vi "Double Point CW.vi"() -> ()   [LabVIEW 2020]
uses:
  Labview Library/Libraries/Basic Experiment/CW Results.ctl
  Labview Library/Libraries/Basic Experiment/CW Fit Frequency.ctl
  <vilib>/Math Plots/2D Math Plots/2D Error Bar/2D Error Bar XCtrl/2D Error Bar.xctl
  <vilib>/Math Plots/2D Math Plots/2D Error Bar/2D Error Bar Datatype/2D Error Bar Datatype.lvclass
  Labview Library/Libraries/Basic Experiment/CW settings.ctl
  Labview Library/Libraries/Basic Experiment/AutoTrace Setting For Exp.ctl
  Labview Library/Libraries/HW_LMMR_ASG8100/LMMR ASG/ASG Instructions XControl.xctl
  <vilib>/Analysis/baseanly.llb/Mean (DBL).vi
  <vilib>/Math Plots/2D Math Plots/2D Error Bar/2D Error Bar Datatype/Public/Plot Helper (Fixed).vi
  <vilib>/express/express arith-compare/Formula/XNode/ExpressFormulaBlockNode.xnode
  Labview Library/Libraries/Basic Experiment/Basic Experiment.lvlib
  Labview Library/Libraries/HW_LMMR_ASG8100/LMMR ASG/ASG 8100 Module.lvlib
  Labview Library/Libraries/HW_NI_CTR/NI DAQ Counter/NI DAQ Counter.lvlib
  <vilib>/Analysis/NI_AALBase.lvlib
  Labview Library/Libraries/HW_Rigol_DSG/Rigol Signal Generator Module/Rigol Signal Generator Module.lvlib
panel:
  in  "?":enum32{"CW Sequence", "CW Spectrum CY", "Check"}(tab)=enum."CW Spectrum CY"
  in  "CW seq":T3(xcontrol)=[{"Flags"=[TRUE, FALSE, FALSE, FALSE, FALSE, FALSE, FALSE, FALSE, FALSE, FALSE, FALSE, FALSE, FALSE, FALSE], "Comments"="", "Time"=2e-06, "Loop Config"={"Loop Code"=enum."Continued", "Number of Loop"=0, "End of Loop"=nan, "Loop Info"=""}}, {"Flags"=[TRUE, FALSE, TRUE, FALSE, FALSE, FALSE, FALSE, FALSE, FALSE, FALSE, FALSE, FALSE, FALSE, FALSE], "Comments"="", "Time"=5e-08, "Loop Config"={"Loop Code"=enum."Continued", "Number of Loop"=0, "End of Loop"=nan, "Loop Info"=""}}, {"Flags"=[TRUE, TRUE, FALSE, FALSE, FALSE, FALSE, FALSE, FALSE, FALSE, FALSE, FALSE, FALSE, FALSE, FALSE], "Comments"="", "Time"=5e-05, "Loop Config"={"Loop Code"=enum."Continued", "Number of Loop"=0, "End of Loop"=nan, "Loop Info"=""}}, {"Flags"=[TRUE, FALSE, TRUE, FALSE, FALSE, FALSE, FALSE, FALSE, FALSE, FALSE, FALSE, FALSE, FALSE, FALSE], "Comments"="", "Time"=5e-08, "Loop Config"={"Loop Code"=enum."Continued", "Number of Loop"=0, "End of Loop"=nan, "Loop Info"=""}}, {"Flags"=[TRUE, FALSE, FALSE, FALSE, FALSE, FALSE, FALSE, FALSE, TRUE, FALSE, FALSE, FALSE, FALSE, FALSE], "Comments"="", "Time"=2e-06, "Loop Config"={"Loop Code"=enum."Continued", "Number of Loop"=0, "End of Loop"=nan, "Loop Info"=""}}, {"Flags"=[TRUE, FALSE, TRUE, FALSE, FALSE, FALSE, FALSE, FALSE, FALSE, FALSE, FALSE, FALSE, FALSE, FALSE], "Comments"="", "Time"=5e-08, "Loop Config"={"Loop Code"=enum."Continued", "Number of Loop"=0, "End of Loop"=nan, "Loop Info"=""}}, {"Flags"=[TRUE, FALSE, FALSE, FALSE, FALSE, FALSE, FALSE, FALSE, FALSE, FALSE, FALSE, FALSE, FALSE, FALSE], "Comments"="", "Time"=5e-05, "Loop Config"={"Loop Code"=enum."Continued", "Number of Loop"=0, "End of Loop"=nan, "Loop Info"=""}}, {"Flags"=[TRUE, FALSE, TRUE, FALSE, FALSE, FALSE, FALSE, FALSE, FALSE, FALSE, FALSE, FALSE, FALSE, FALSE], "Comments"="", "Time"=5e-08, "Loop Config"={"Loop Code"=enum."Continued", "Number of Loop"=0, "End of Loop"=nan, "Loop Info"=""}}, {"Flags"=[TRUE, FALSE, FALSE, FALSE, FALSE, FALSE, FALSE, FALSE, FALSE, FALSE, FALSE, FALSE, FALSE, FALSE], "Comments"="", "Time"=2e-06, "Loop Config"={"Loop Code"=enum."Continued", "Number of Loop"=0, "End of Loop"=nan, "Loop Info"=""}}]
  out "Signal and Ref 2":cluster{"Numeric":dbl, "Numeric":dbl}(graph)={"Numeric"=11988.666666666666, "Numeric"=11908.666666666666}
  out "Signal and Ref":cluster{"Numeric":dbl, "Numeric":dbl}(graph)={"Numeric"=12031.333333333334, "Numeric"=11977.333333333332}
  in  "Settings":T4={"Num Pts"=10000, "Start freq"=1367.0, "Stop freq"=1373.0, " dBm"=-7.0, "Ratio \nThre(abs)"=0.03, "AutoTrace Before Exp"=FALSE, "RepoSave"=FALSE, "Peak Num \nLimit "=2, "Loop per Update"=1200, "UpdateTime"=25} {"UpdateTime" format="%.0p"; "Loop per Update" format="%#_6p"}
  in  "AutoTrace Settings":T5={"Ratio"=0.5, "Threshold"=7170.999999999999, "Trace Times"=0, "Max Times"=100, "AutoTrace Status"=enum."Normal"}
  out "Total Time (min)":ext=1062.1593 format="%#.5p"
  out "Readout Result":refnum<class "2D Plot Datatype.lvclass">[](xcontrol) caption="2D Error Bar"
  out "CW Result":T6={"Fit Frequency"={"Fre2"={"Amplitude"=nan, "Position"=nan, "Width"=nan}, "Fre1"={"Amplitude"=nan, "Position"=nan, "Width"=nan}, "Fre3"={"Amplitude"=nan, "Position"=nan, "Width"=nan}, "Background"=0.0}, "Pro"=[], "Error Bar"=[0.009618072395389447, 0.010023899080911879, 0.0099506405925294, 0.010065376148420763, 0.010199717043787939, 0.010260847634534493, 0.010058201169096073, 0.010330373101194222, 0.010347960338142663, 0.010432270152347089, 0.010424891842338956, 0.010339921852896642, 0.01058656495840666, 0.010634567325262224], "Raw Data Path"=path "", "Image Path"=path ""}
  out "Pro Array":dbl[](array[numeric])=[-0.0022504507719500744, 0.003304738238140814, -0.01707959605598075, -0.01598738795963195, -0.00726438373136129, -0.005972380429531077, -0.030821164777634635, -0.009807610308887105, -0.011284996490708799, -0.006280515739338632, -0.0033235649624780983, -0.010049154116550496, 0.006197937645131102, 0.007759603066543885]
  in  "error in (no error)":errorcluster={"status"=FALSE, "code"=1073676294, "source"="VISA Read in YP60.lvlib:Wrap VISA Read.vi:5740004->YP60.lvlib:VISA Set Current.vi:2010003->YP60.lvlib:Set Core.vi->YP60.lvlib:Main.vi"}
  out "error out":errorcluster={"status"=TRUE, "code"=-1073807194, "source"="VISA Write in Rigol Signal Generator Module.lvlib:Stop - CORE.vi->Rigol Signal Generator Module.lvlib:Main.vi->Rigol Signal Generator Module.lvlib:Main.vi.ACBRProxyCaller.FA10008D"}
  # "CW Settings"
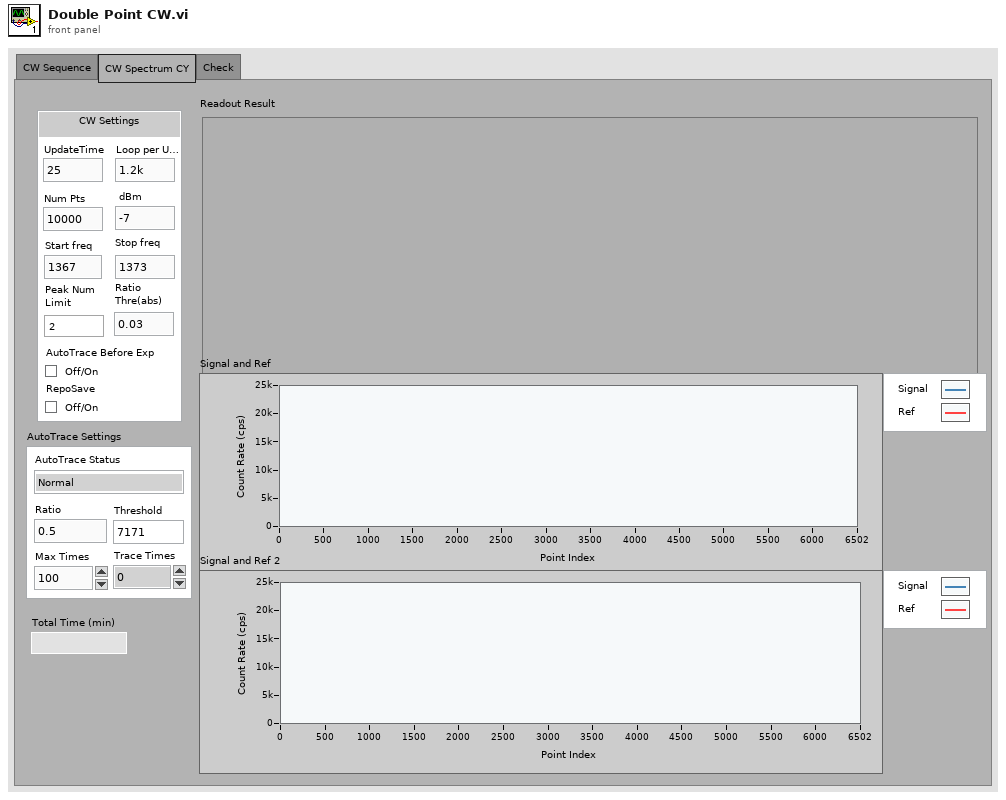
[diagram p1: front panel]
types:
  T1 = typedef "Loop XControl.xctl/Loop Config.ctl" = cluster{"Loop Code":T2, "Number of Loop":i32, "End of Loop":dbl, "Loop Info":string}
  T2 = typedef "Loop XControl.xctl/Loop Code.ctl" = enum16{"Continued", "Loop", "End Loop"}
  T3 = cluster{"Flags":bool[], "Comments":string, "Time":dbl, "Loop Config":T1}[]
  T4 = typedef "Basic Experiment.lvlib/CW settings.ctl" = cluster{"Num Pts":i32, "Start freq":dbl, "Stop freq":dbl, " dBm":dbl, "Ratio \nThre(abs)":dbl, "AutoTrace Before Exp":bool, "RepoSave":bool, "Peak Num \nLimit ":i32, "Loop per Update":u32, "UpdateTime":i32}
  T5 = typedef "Basic Experiment.lvlib/AutoTrace Setting For Exp.ctl" = cluster{"Ratio":dbl, "Threshold":dbl, "Trace Times":i32, "Max Times":i32, "AutoTrace Status":enum16{"Normal", "AutoTrace  Last Loop", "Unintialized"}}
  T6 = typedef "Basic Experiment.lvlib/CW Results.ctl" = cluster{"Fit Frequency":T7, "Pro":dbl[], "Error Bar":dbl[], "Raw Data Path":path, "Image Path":path}
  T7 = typedef "Basic Experiment.lvlib/CW Fit Frequency.ctl" = cluster{"Fre2":cluster{"Amplitude":dbl, "Position":dbl, "Width":dbl}, "Fre1":cluster{"Amplitude":dbl, "Position":dbl, "Width":dbl}, "Fre3":cluster{"Amplitude":dbl, "Position":dbl, "Width":dbl}, "Background":dbl}
  T8 = cluster{"Sweep Amplitude (V)":dbl, "Freq Start (Hz)":dbl, "Freq Stop (Hz)":dbl, "Num of Point":i32}
  T9 = enum16{"Normal", "AutoTrace  Last Loop", "Unintialized"}
  T10 = enum16{"open", "open or create", "create or replace", "create", "open (read-only)"}
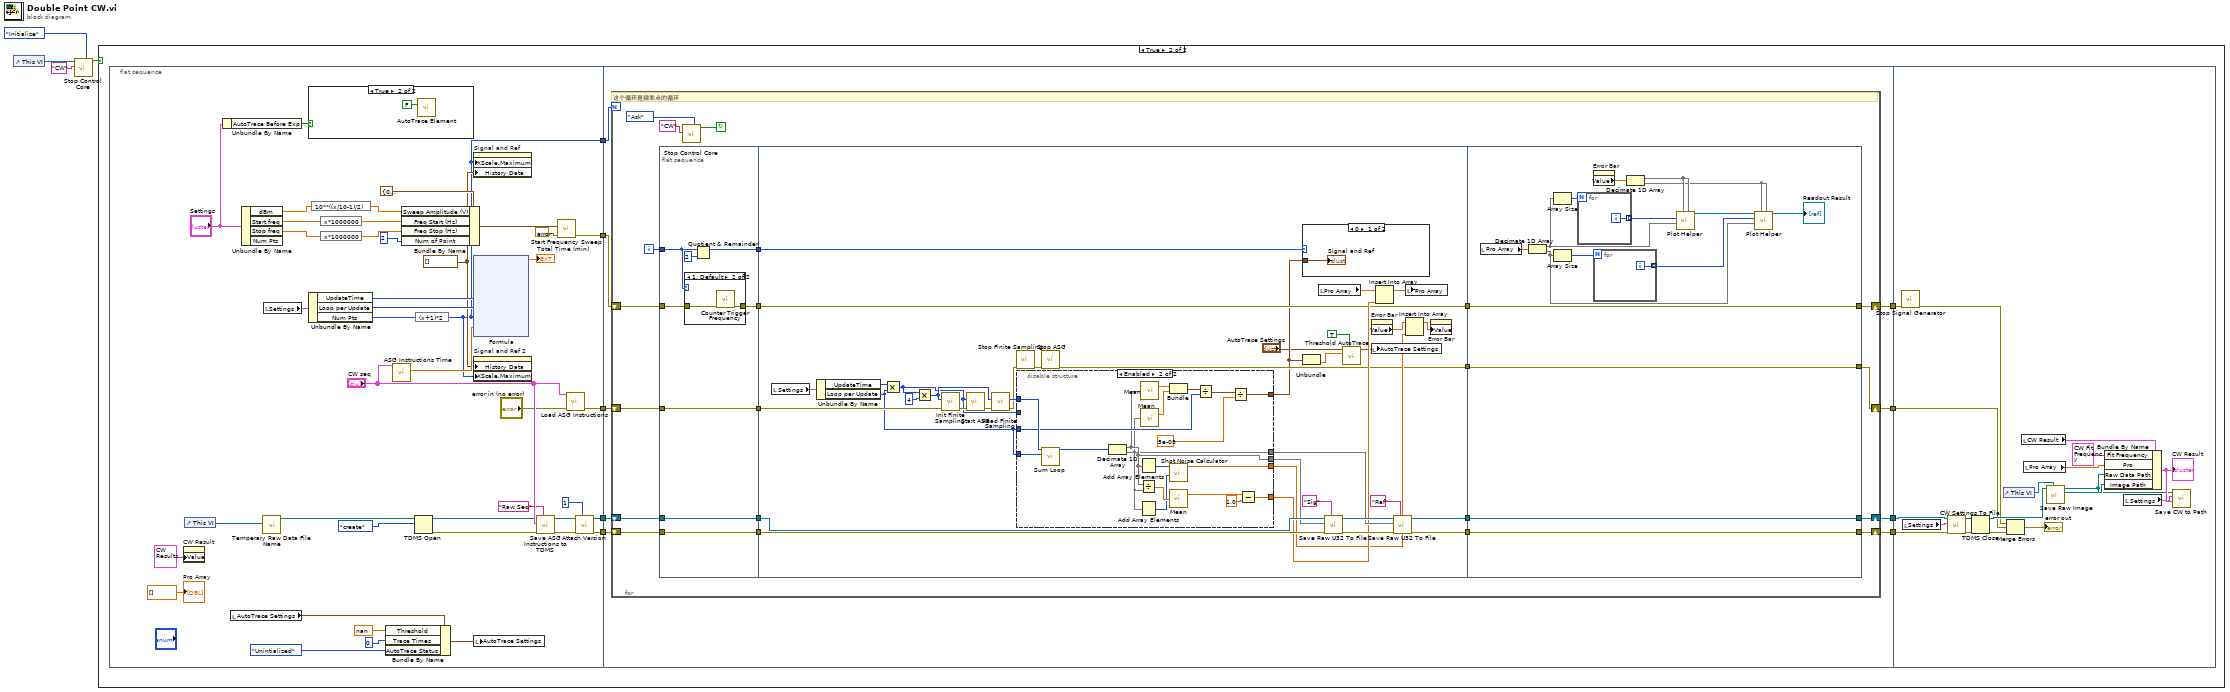
[diagram p0: block diagram]
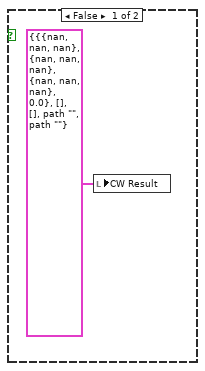
[diagram p2: hidden frame]
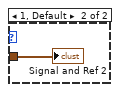
[diagram p5: hidden frame]
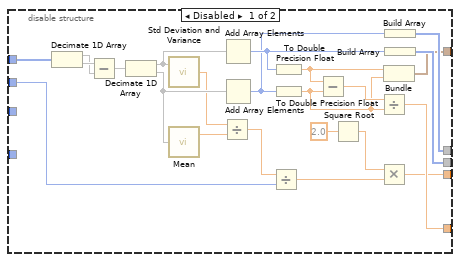
[diagram p6: hidden frame]
diagram:
  n1 = control-ref of="This VI"() -> (w3:refnum<vi>)
  n2 = call "Stop Control Core.vi"("Mode"=enum16{"Ask", "Initialize"}."Initialize", "Program Name"="CW", "VI Ref"=w3) -> ("Continue Sign(Continue:True)"=w1:bool)  [unwired: 8 in]
  n3 = case shown="True" w1 {
    frame False {
      n4 = local write "CW Result"(T6 {"Fit Frequency"={"Fre2"={"Amplitude"=nan, "Position"=nan, "Width"=nan}, "Fre1"={"Amplitude"=nan, "Position"=nan, "Width"=nan}, "Fre3"={"Amplitude"=nan, "Position"=nan, "Width"=nan}, "Background"=0.0}, "Pro"=[], "Error Bar"=[], "Raw Data Path"=path "", "Image Path"=path ""} ("CW Result")) -> ()
    }
    frame True {
      n5 = flat-sequence {
        tunnel: [w35] -> w11
        tunnel: [w39] -> w10
        tunnel: [w38] -> w9
        tunnel: [w37] -> w8
        tunnel: [w16] -> w6
        tunnel: [w80] -> w14
        tunnel: [w79] -> w13
        tunnel: [w78] -> w12
        tunnel: w11 -> [w77]
        tunnel: w10 -> [w76]
        tunnel: w9 -> [w75]
        tunnel: w8 -> [w74]
        tunnel: [w73] -> w7
        tunnel: w6 -> [w72]
        tunnel: w14 -> [w229]
        tunnel: w13 -> [w228]
        tunnel: w12 -> [w216]
        tunnel: w7 -> [w214]
        frame #0 {
          w17 = cluster{"Signal":dbl, "Ref":dbl}[] [] ("History Data")
          n6 = property on="CW Result" class="Clust (strict)"("Value"=T6 {"Fit Frequency"={"Fre2"={"Amplitude"=nan, "Position"=nan, "Width"=nan}, "Fre1"={"Amplitude"=nan, "Position"=nan, "Width"=nan}, "Fre3"={"Amplitude"=nan, "Position"=nan, "Width"=nan}, "Background"=0.0}, "Pro"=[], "Error Bar"=[], "Raw Data Path"=path "", "Image Path"=path ""} ("CW Result")) -> ()  [unwired: 2 in, 2 out]
          n7 = control-ref of="This VI"() -> (w43:refnum<vi>)
          n8 = Unbundle By Name("Settings") -> ("AutoTrace Before Exp"=w55:bool)
          n9 = local read "AutoTrace Settings"() -> (w15:T5)
          n10 = Unbundle By Name("Settings") -> ("dBm"=w52:dbl, "Start freq"=w31:dbl, "Stop freq"=w30:dbl)  [unwired: 1 out]
          n11 = call "Temperary Raw Data File Name.vi"("VI ref"=w43) -> ("Raw data Path"=w44:path)  [unwired: 10 in]
          n12 = local read "Settings"() -> (w48:T4)
          n13 = case shown="True" w55 {
            frame False {
            }
            frame True {
              n14 = call "AutoTrace Element.vi"("Need Correct Count?(T)"=FALSE) -> ()  [unwired: 9 in, 2 out]
            }
          }
          n15 = Unbundle By Name(w48) -> ("UpdateTime"=w26:i32, "Loop per Update"=w25:u32, "Num Pts"=w22:i32)
          n16 = expression code="10**((x/10-1)/2)"(w52) -> (w33:dbl)
          n17 = expression code="x*1000000"(w31) -> (w29:dbl)
          n18 = expression code="x*1000000"(w30) -> (w28:dbl)
          n19 = Bundle By Name(cluster=w15, "Threshold"=nan, "Trace Times"=0, "AutoTrace Status"=T9."Unintialized" ("Value")) -> (w18:T5)
          n20 = call "ASG Instructions Time.vi"("ASG Instr. A"="CW seq") -> ("Total Time (s)"=w24:ext)  [unwired: 10 in]
          n21 = Bundle By Name(cluster=T8 {"Sweep Amplitude (V)"=0.01, "Freq Start (Hz)"=2865000000.0, "Freq Stop (Hz)"=2875000000.0, "Num of Point"=10} ("Frequency Sweep Configure"), "Sweep Amplitude (V)"=w33, "Freq Start (Hz)"=w29, "Freq Stop (Hz)"=w28, "Num of Point"=2) -> (w27:T8)
          n22 = TDMS Open(10:T10."create" ("operation (0:open)"), 11:w44) -> (0:w46:errorcluster, 3:w45:refnum<k34>)  [unwired: 5 in]
          n23 = expression code="(x+1)*2"(w22) -> (w16:i32)
          n24 = property on="Signal and Ref" class="WFChart (strict)"("XScale.Maximum"=w16, "History Data"=w17) -> ()  [unwired: 2 in, 2 out]
          n25 = xnode "Formula"("Update Time"=w26, "Loop per Update"=w25, "Num Pts"=w16, "Seq Time"=w24) -> ("Result"=→"Total Time (min)":ext)  [unwired: 1 in, 1 out]
          n26 = property on="Signal and Ref 2" class="WFChart (strict)"("History Data"=w17, "XScale.Maximum"=w16) -> ()  [unwired: 2 in, 2 out]
          n27 = local write "AutoTrace Settings"(w18) -> ()
          n28 = call "Save ASG Instructions to TDMS.vi"("Name"="Raw Seq", "error in (no error)"=w46, "ASG Instructions"="CW seq", "tdms file"=w45) -> ("error out"=w51:errorcluster, "tdms file out"=w50:refnum<k34>)  [unwired: 6 in]
          n29 = call "Start Frequency Sweep.vi"("error in"=errorcluster {"status"=FALSE, "code"=0, "source"=""}, "Frequency Sweep Configure"=w27) -> ("error out"=w35:errorcluster)  [unwired: 8 in, 1 out]
          n30 = call "Load ASG Instructions.vi"("error in (no error)"="error in (no error)", "ASG Instructions"="CW seq") -> ("error out"=w39:errorcluster)  [unwired: 9 in]
          n31 = call "Attach Version.vi"("Version"=u32 1, "error in (no error)"=w51, "Refnum in"=w50) -> ("error out"=w38:errorcluster, "Refnum out"=w37:refnum<k34>)  [unwired: 5 in, 2 out]
          "Pro Array" <- dbl[] [] ("Pro Array")
        }
        frame #1 {
          n32 = for {
            N: w72 -> [_]
            shift-right: [w97] -> w79
            shift-left: w75 -> [w100]
            shift-right: [w98] -> w80
            shift-left: w74 -> [w96]
            shift-right: [w86] -> w78
            shift-left: w77 -> [w89]
            shift-right: [w82] -> w73
            shift-left: w76 -> [w84]
            i -> [w85]
            stop <- w93 continue-if-true
            # "这个循环是频率点的循环"
            n33 = flat-sequence {
              tunnel: w96 -> [w109]
              tunnel: [w109] -> w101
              tunnel: w100 -> [w108]
              tunnel: [w108] -> w99
              tunnel: [w105] -> w90
              tunnel: w89 -> [w107]
              tunnel: [w106] -> w87
              tunnel: w85 -> [w104]
              tunnel: w84 -> [w105]
              tunnel: [w102] -> w81
              tunnel: w99 -> [w138]
              tunnel: w101 -> [w139]
              tunnel: [w134] -> w92
              tunnel: [w136] -> w91
              tunnel: w90 -> [w122]
              tunnel: [w120] -> w88
              tunnel: w87 -> [w120]
              tunnel: [w119] -> w83
              tunnel: w81 -> [w118]
              tunnel: [w207] -> w97
              tunnel: [w208] -> w98
              tunnel: w92 -> [w208]
              tunnel: w91 -> [w207]
              tunnel: [w206] -> w86
              tunnel: w88 -> [w206]
              tunnel: w83 -> [w205]
              tunnel: [w205] -> w82
              frame #0 {
                n34 = case shown="1, Default" w104 {
                  tunnel: w107 -> [w110 w112]
                  tunnel: [w110 w111] -> w106
                  frame 0 {
                  }
                  frame 1, Default {
                    n35 = call "Counter Trigger Frequency.vi"("error in"=w112) -> ("error out"=w111:errorcluster)  [unwired: 9 in, 1 out]
                  }
                }
                n36 = Quotient & Remainder(x=w104, y=2) -> (x-y*floor(x/y)=w102:i32)  [unwired: 1 out]
              }
              frame #1 {
                n37 = local read "Settings"() -> (w131:T4)
                n38 = Unbundle By Name(w131) -> ("UpdateTime"=w123:i32, "Loop per Update"=w121:u32)
                n39 = Multiply(x=w123, y=w121) -> (x*y=w124:u32)
                n40 = Multiply(x=w124, y=4) -> (x*y=w144:u32)
                n41 = call "Init Finite Sampling.vi"("error in"=w122, "Num of Sample"=w144) -> ("error out"=w141:errorcluster)  [unwired: 9 in]
                n42 = call "Start ASG.vi"("error in (no error)"=w141, "Loop Number"=w124) -> ("error out"=w140:errorcluster)  [unwired: 8 in, 1 out]
                n43 = call "Read Finite Sampling.vi"("error in"=w140, "Samples to Read"=w144) -> ("error out"=w145:errorcluster, "Sample Array"=w148:u32[])  [unwired: 7 in, 1 out]
                n44 = call "Stop Finite Sampling.vi"("error in"=w145) -> ("error out"=w142:errorcluster)  [unwired: 10 in]
                n45 = disable-structure shown="Enabled" {
                  disable-tunnel: w148 -> [w171 w192]
                  disable-tunnel: w121 -> [_ w191]
                  disable-tunnel: [w166 w178] -> w128
                  disable-tunnel: [w165 w177] -> w127
                  disable-tunnel: [w162 w186] -> w126
                  disable-tunnel: w124 -> [w154 _]
                  disable-tunnel: [w152 w174] -> w125
                  disable-tunnel: [w151 w179] -> w117
                  disable-tunnel: w121 -> [_ w182]
                  frame Disabled {
                    n46 = Decimate 1D Array(w171) -> (w172:u32[], w173:u32[])
                    n47 = Subtract(x=w173, y=w172) -> (x-y=w170:u32[])
                    n48 = Decimate 1D Array(w170) -> (w167:u32[], w164:u32[])
                    n49 = call <vilib>:"Std Deviation and Variance.vi"("X"=w167) -> ("standard deviation"=w156:dbl)  [unwired: 1 in, 2 out]
                    n50 = call-poly <vilib>:"Mean.vi"("X"=w164) -> ("mean"=w153:dbl)  [unwired: 1 out]
                    n51 = Divide(x=w156, y=w153) -> (x/y=w157:dbl)
                    n52 = Add Array Elements(numeric array=w167) -> (sum=w169:u32)
                    n53 = Add Array Elements(numeric array=w164) -> (sum=w168:u32)
                    n54 = Divide(x=w157, y=w154) -> (x/y=w159:dbl)
                    n55 = To Double Precision Float(number=w169) -> (double precision float=w160:dbl)
                    n56 = To Double Precision Float(number=w168) -> (double precision float=w161:dbl)
                    n57 = Subtract(x=w160, y=w161) -> (x-y=w163:dbl)
                    n58 = Square Root(x=2.0) -> (sqrt(x)=w158:dbl)
                    n59 = Divide(x=w163, y=w161) -> (x/y=w162:dbl)
                    n60 = Multiply(x=w158, y=w159) -> (x*y=w152:dbl)
                    n61 = Bundle(w160, w161) -> (w151:cluster{dbl, dbl})  [unwired: 1 in]
                    n62 = Build Array(w168) -> (w165:u32[])
                    n63 = Build Array(w169) -> (w166:u32[])
                  }
                  frame Enabled {
                    n64 = call "Sum Loop.vi"("Loop per Update"=w191, "Raw Data Array"=w192) -> ("Data after sum"=w190:u32[])  [unwired: 9 in]
                    n65 = Decimate 1D Array(w190) -> (w178:u32[], w177:u32[])
                    n66 = Add Array Elements(numeric array=w178) -> (sum=w176:u32)
                    n67 = Divide(x=w178, y=w177) -> (x/y=w189:dbl[])
                    n68 = Add Array Elements(numeric array=w177) -> (sum=w175:u32)
                    n69 = call-poly <vilib>:"Mean.vi"("X"=w178) -> ("mean"=w185:dbl)  [unwired: 1 out]
                    n70 = call-poly <vilib>:"Mean.vi"("X"=w177) -> ("mean"=w184:dbl)  [unwired: 1 out]
                    n71 = Bundle("mean"=w185, "mean"=w184) -> (w183:cluster{"mean":dbl, "mean":dbl})  [unwired: 1 in]
                    n72 = call "Shot Noise Calculator.vi"("Toral Ref Count"=w175, "Total Sig Count"=w176) -> ("Error Given By ShotNoise"=w174:dbl)  [unwired: 9 in]
                    n73 = call-poly <vilib>:"Mean.vi"("X"=w189) -> ("mean"=w188:dbl)  [unwired: 1 out]
                    n74 = Divide(x=w183, y=w182) -> (x/y=w181:cluster{"mean":dbl, "mean":dbl})
                    n75 = Divide(x=w181, y=5e-05) -> (x/y=w179:cluster{"mean":dbl, "mean":dbl})
                    n76 = Subtract(x=w188, y=1.0) -> (x-y=w186:dbl)
                  }
                }
                n77 = call "Stop ASG.vi"("error in (no error)"=w142) -> ("error out"=w119:errorcluster)  [unwired: 9 in, 1 out]
                n78 = case shown="0" w118 {
                  tunnel: w117 -> [w149 w150]
                  frame 0 {
                    "Signal and Ref" <- w149
                  }
                  frame 1, Default {
                    "Signal and Ref 2" <- w150
                  }
                }
                n79 = Unbundle(w117) -> ("mean"=w113:dbl)  [unwired: 1 out]
                n80 = local read "Pro Array"() -> (w147:dbl[])
                n81 = call "Save Raw U32 To File.vi"("Suffix"="Sig" ("PS"), "error in"=w138, "Sample Array"=w128, "Refnum in"=w139) -> ("error out"=w137:errorcluster, "tdms file out"=w135:refnum<k34>)  [unwired: 4 in, 2 out]
                n82 = call "Threshold AutoTrace.vi"("Play Sequence"=TRUE, "Count"=w113, "AutoTrace Settings In"="AutoTrace Settings") -> ("AutoTrace Settings Out"=w115:T5)  [unwired: 7 in, 1 out]
                n83 = property on="Error Bar" class="Arr (strict)"() -> ("Value"=w133:dbl[])  [unwired: 2 in, 2 out]
                n84 = local write "AutoTrace Settings"(w115) -> ()
                n85 = Insert Into Array(array=w147, new element=w126) -> (w146:dbl[])  [unwired: 1 in]
                n86 = call "Save Raw U32 To File.vi"("Suffix"="Ref" ("PS"), "error in"=w137, "Sample Array"=w127, "Refnum in"=w135) -> ("error out"=w136:errorcluster, "tdms file out"=w134:refnum<k34>)  [unwired: 4 in, 2 out]
                n87 = local write "Pro Array"(w146) -> ()
                n88 = Insert Into Array(array=w133, new element=w125) -> (w132:dbl[])  [unwired: 1 in]
                n89 = property on="Error Bar" class="Arr (strict)"("Value"=w132) -> ()  [unwired: 2 in, 2 out]
              }
              frame #2 {
                n90 = local read "Pro Array"() -> (w196:dbl[])
                n91 = Decimate 1D Array(w196) -> (w195:dbl[], w194:dbl[])
                n92 = Array Size(array=w195) -> (size(s)=w204:i32)
                n93 = Array Size(array=w194) -> (size(s)=w200:i32)
                n94 = for {
                  N: w204 -> [_]
                  tunnel: [w210] -> w203 mode=indexing
                  i -> [w210]
                }
                n95 = property on="Error Bar" class="Arr (strict)"() -> ("Value"=w199:dbl[])  [unwired: 2 in, 2 out]
                n96 = for {
                  N: w200 -> [_]
                  tunnel: [w209] -> w193 mode=indexing
                  i -> [w209]
                }
                n97 = Decimate 1D Array(w199) -> (w198:dbl[], w197:dbl[])
                n98 = call-poly <vilib>:"Plot Helper.vi"("error b vector"=w198, "error a vector"=w198, "y vector"=w195, "x vector"=w203) -> ("2D Plot Class Obj Array out"=w202:refnum<class "2D Plot Datatype.lvclass">[])  [unwired: 2 in, 5 out]
                n99 = call-poly <vilib>:"Plot Helper.vi"("error b vector"=w197, "error a vector"=w197, "y vector"=w194, "x vector"=w193, "2D Plot Class Obj Array in"=w202) -> ("2D Plot Class Obj Array out"=→"Readout Result":refnum<class "2D Plot Datatype.lvclass">[])  [unwired: 1 in, 5 out]
              }
            }
            n100 = call "Stop Control Core.vi"("Mode"=enum16{"Ask", "Initialize"}."Ask", "Program Name"="CW") -> ("Continue Sign(Continue:True)"=w93:bool)  [unwired: 9 in]
          }
        }
        frame #2 {
          n101 = call "Stop Signal Generator.vi"("error in"=w216) -> ("error out"=w213:errorcluster)  [unwired: 9 in, 1 out]
          n102 = local read "Settings"() -> (w217:T4)
          n103 = call "CW Settings To File.vi"("error in (no error)"=w228, "CW settings"=w217, "tdms file"=w229) -> ("error out"=w226:errorcluster, "tdms file out"=w227:refnum<k34>)  [unwired: 7 in]
          n104 = TDMS Close(8:w226, 11:w227) -> (0:w212:errorcluster, 3:w224:path)
          n105 = control-ref of="This VI"() -> (w225:refnum<vi>)
          n106 = Merge Errors(w213, w214, w212) -> (→"error out":errorcluster)
          n107 = local read "CW Result"() -> (w218:T6)
          n108 = local read "Pro Array"() -> (w223:dbl[])
          n109 = call "Save Raw Image.vi"("reference"=w225, "Raw TDMS Path"=w224) -> ("Image Path"=w222:path, "Raw TDMS Path Out"=w219:path)  [unwired: 7 in, 1 out]
          n110 = Bundle By Name(cluster=w218, "Fit Frequency"=T7 {"Fre2"={"Amplitude"=nan, "Position"=nan, "Width"=nan}, "Fre1"={"Amplitude"=nan, "Position"=nan, "Width"=nan}, "Fre3"={"Amplitude"=nan, "Position"=nan, "Width"=nan}, "Background"=0.0}, "Pro"=w223, "Raw Data Path"=w219, "Image Path"=w222) -> (w221:T6)
          "CW Result" <- w221
          n111 = local read "Settings"() -> (w220:T4)
          n112 = call "Save CW to Path.vi"("CW Result"=w221, "setting section"=w220, "file path"=w219) -> ()  [unwired: 5 in, 4 out]
        }
      }
    }
  }
